vi "FGV_DOCK_REPORT_records_display.vi"(7 "options":T1, 8 "error_in":errorcluster, 11 "input":variant) -> (0 "error_out":errorcluster, 3 "output":variant)   [LabVIEW 2019]
uses:
  FGV_DOCK_REPORT_records_display.ctl
  DOCK_REPORT_references.ctl
  DOCK_REPORT_all_info.ctl
  SQL_CLIENT/MAIN/REPORTS/DATES/typedef/REPORT_DATES_statuses.ctl
  _misc/AULocalize/SubVIs/Get Localized Phrase Compact Interface 1D.vi
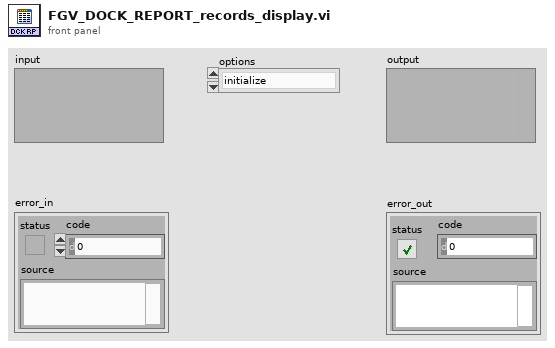
[diagram p1: front panel]
types:
  T1 = typedef "FGV_DOCK_REPORT_records_display.ctl" = enum16{"initialize", "set_cbatch_code", "set_records", "display", "clear", "get_all_info"}
  T2 = typedef "DOCK_REPORT_all_info.ctl" = cluster{"batch_code":string, "records":string[][], "record_statuses":T3[], "column_headers":string[], "column_widths":i16[], "DOCK_REPORT_references":T4}
  T3 = typedef "REPORT_DATES_statuses.ctl" = enum16{"GEAR_OK", "GEAR_NOK", "GEAR_interrupted", "GEAR_in_operation", "GEAR_unexpected"}
  T4 = typedef "DOCK_REPORT_references.ctl" = cluster{"front_panel_reference":refnum<vi>, "SQL_listbox_reference":refnum<vi>}
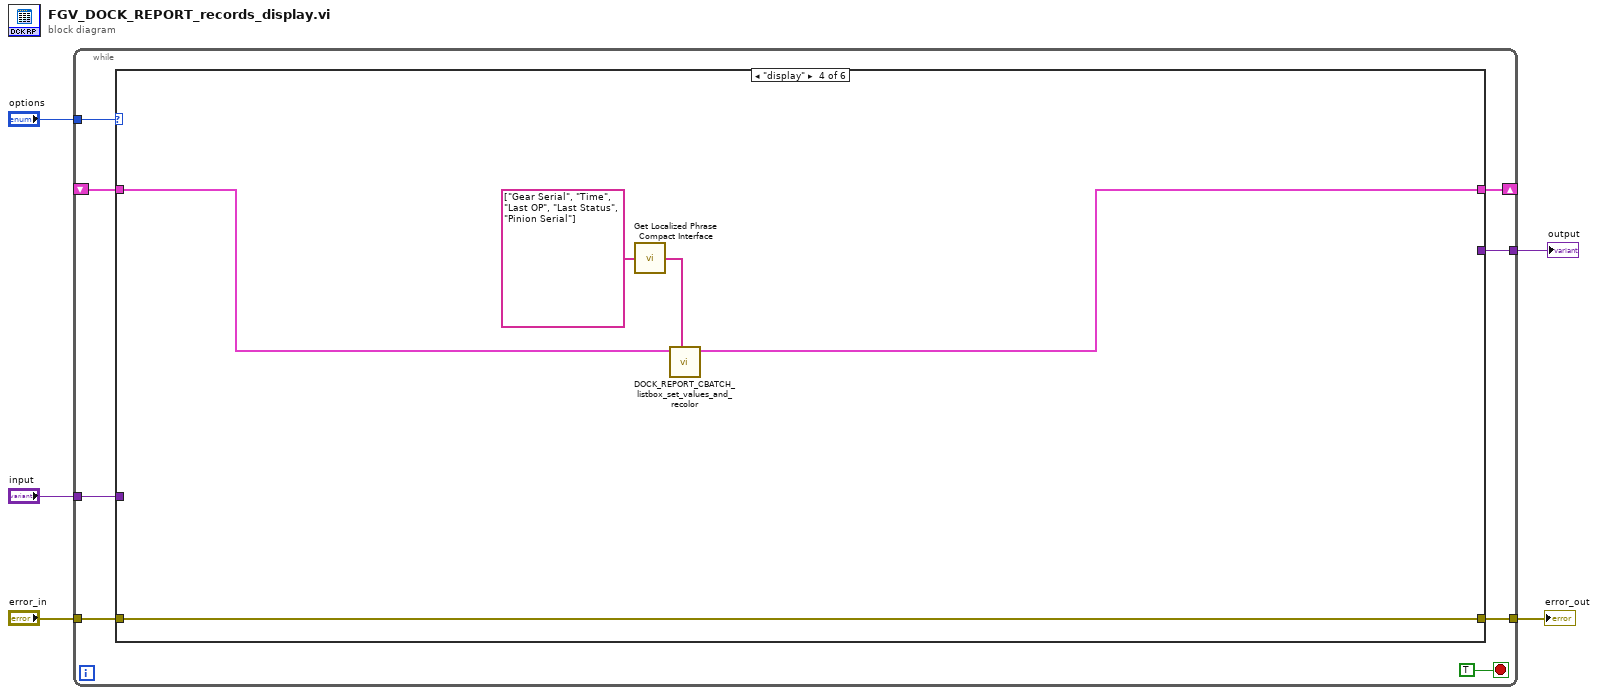
[diagram p0: block diagram]
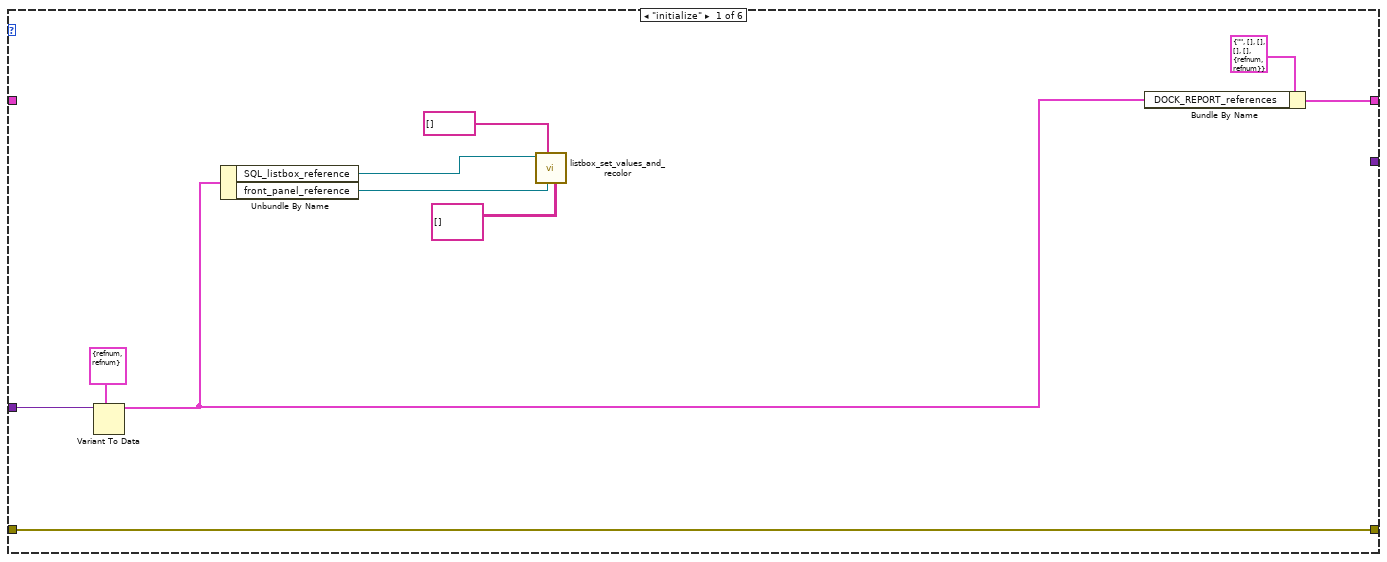
[diagram p2: hidden frame]
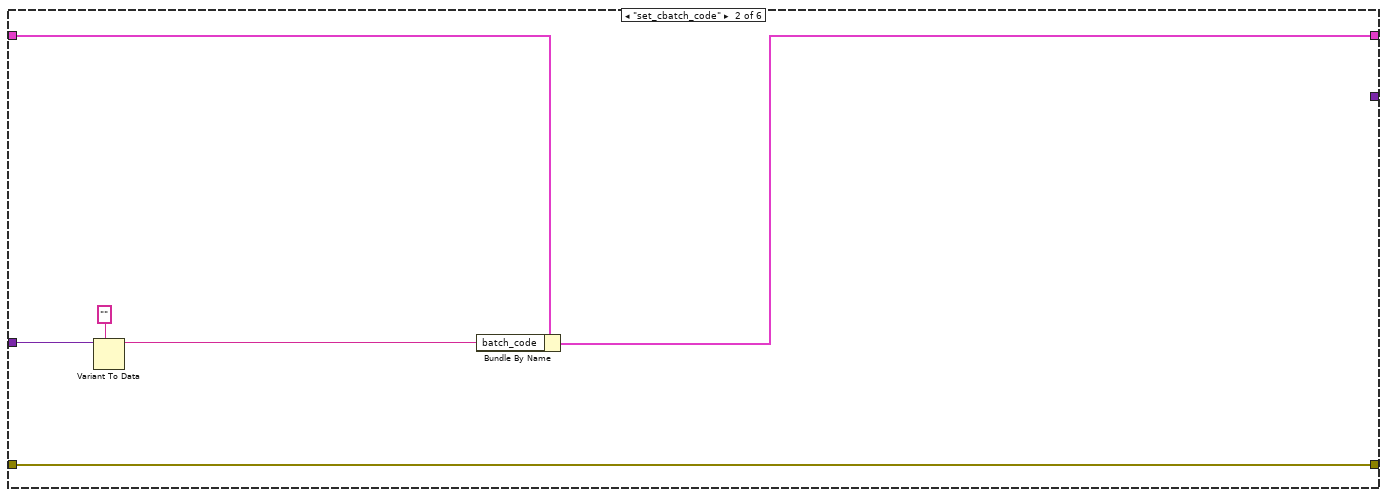
[diagram p3: hidden frame]
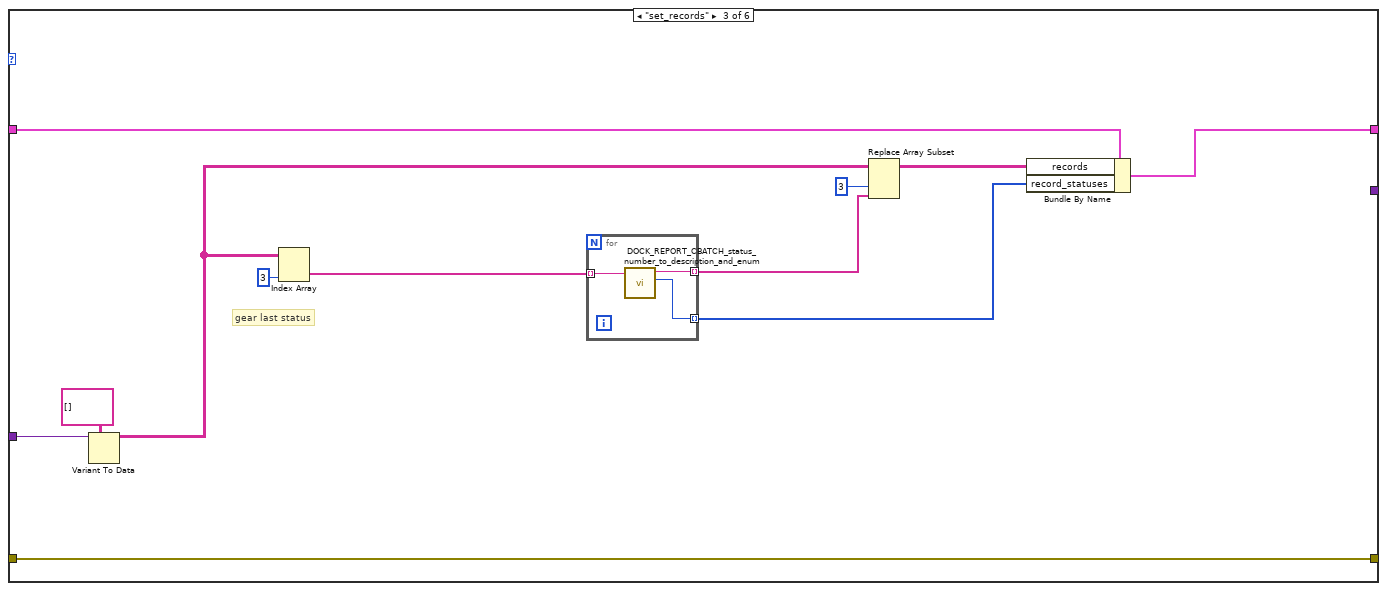
[diagram p4: hidden frame]
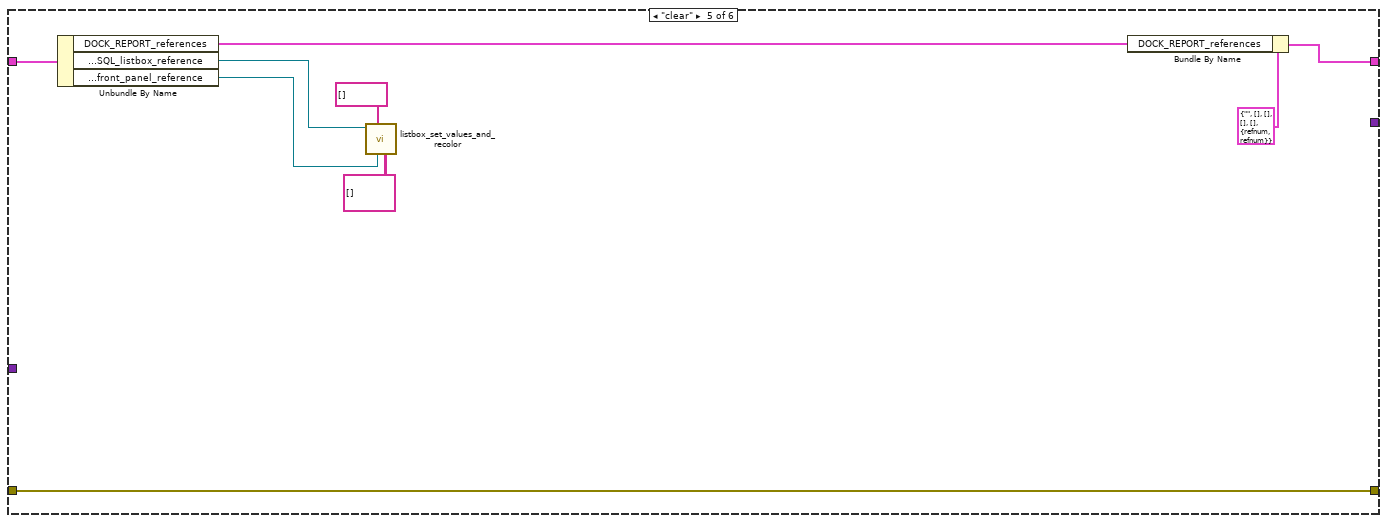
[diagram p5: hidden frame]
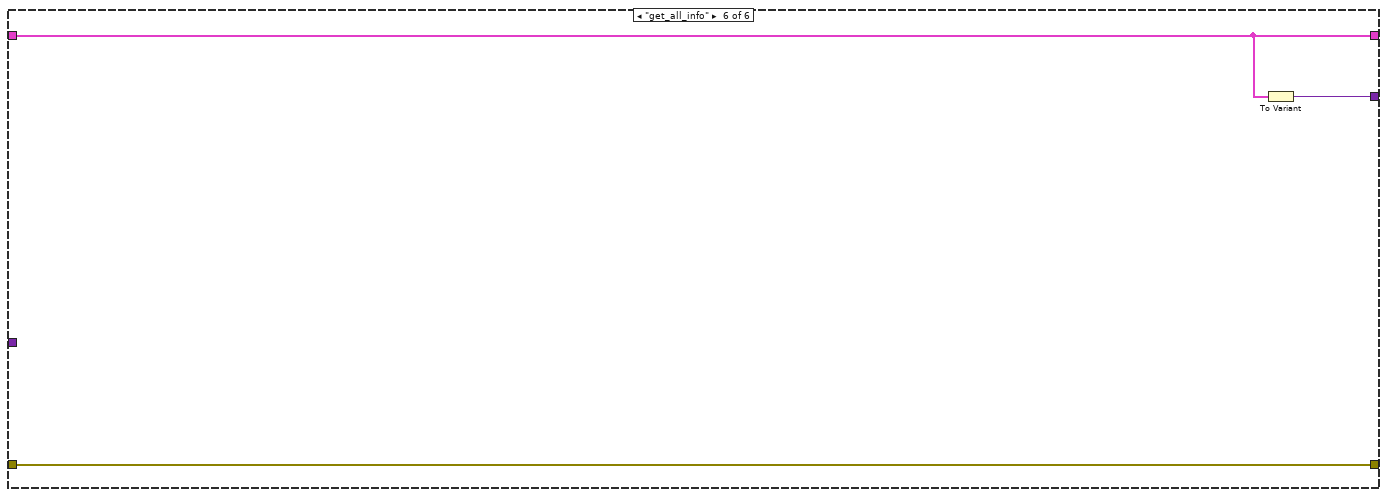
[diagram p6: hidden frame]
diagram:
  n1 = while {
    tunnel: "options" -> [w12]
    tunnel: [w11] -> w5
    tunnel: "error_in" -> [w10]
    shift-right: [w9] -> _
    shift-left: _ -> [w8]
    tunnel: "input" -> [w7]
    tunnel: [w6] -> w1
    stop <- TRUE stop-if-true
    n2 = case shown="\"display\"" w12 {
      tunnel: [w23 w24 w30 w49 w58 w61] -> w11
      tunnel: w10 -> [w23 w24 w30 w49 w58 w61]
      tunnel: [w15 w25 w31 w46 w52 w59] -> w9
      tunnel: w8 -> [_ w26 w32 w47 w55 w59]
      tunnel: w7 -> [w19 w27 w33 _ _ _]
      tunnel: [_ _ _ _ _ w60] -> w6
      frame "initialize" {
        n3 = Variant To Data(type=T4 {"front_panel_reference"=refnum, "SQL_listbox_reference"=refnum} ("REWORK_references"), Variant=w19) -> (data=w16:T4)  [unwired: 1 in, 1 out]
        n4 = Unbundle By Name(w16) -> ("SQL_listbox_reference"=w17:refnum<vi>, "front_panel_reference"=w18:refnum<vi>)
        n5 = call "listbox_set_values_and_recolor.vi"("item_names"=string[][] [], "front_panel_reference"=w18, "column_names"=string[] [], "multicolumn_listbox_reference_in"=w17) -> ()  [unwired: 6 in, 2 out]
        n6 = Bundle By Name(cluster=T2 {"batch_code"="", "records"=[], "record_statuses"=[], "column_headers"=[], "column_widths"=[], "DOCK_REPORT_references"={"front_panel_reference"=refnum, "SQL_listbox_reference"=refnum}} ("REPORT_all_info"), "DOCK_REPORT_references"=w16) -> (w15:T2)
      }
      frame "set_cbatch_code" {
        n7 = Variant To Data(type="", Variant=w27) -> (data=w28:string)  [unwired: 1 in, 1 out]
        n8 = Bundle By Name(cluster=w26, "batch_code"=w28) -> (w25:T2)
      }
      frame "set_records" {
        # "gear last status"
        n9 = Variant To Data(type=string[][] [], Variant=w33) -> (data=w37:string[][])  [unwired: 1 in, 1 out]
        n10 = Index Array(array=w37, index (col)=3 ("disabled index (col)")) -> (element=w39:string[])  [unwired: 1 in]
        n11 = for {
          tunnel: w39 -> [w44] mode=indexing
          tunnel: [w43] -> w38 mode=indexing
          tunnel: [w42] -> w34 mode=indexing
          n12 = call "DOCK_REPORT_CBATCH_status_number_to_description_and_enum.vi"("status_nmb"=w44) -> ("status_enum"=w43:T3, "status_description"=w42:string)  [unwired: 9 in]
        }
        n13 = Replace Array Subset(array=w37, new element=w34, index (col)=3 ("disabled index (col)")) -> (w35:string[][])  [unwired: 1 in]
        n14 = Bundle By Name(cluster=w32, "records"=w35, "record_statuses"=w38) -> (w31:T2)
      }
      frame "display" {
        n15 = call-poly "Get Localized Phrase Compact Interface.vi"("Key"=string[] ["Gear Serial", "Time", "Last OP", "Last Status", "Pinion Serial"] ("column_names")) -> ("Translated Phrase"=w45:string[])
        n16 = call "DOCK_REPORT_CBATCH_listbox_set_values_and_recolor.vi"("column_names"=w45, "REPORT_all_info_in"=w47) -> ("REPORT_all_info_out"=w46:T2)  [unwired: 8 in, 1 out]
      }
      frame "clear" {
        n17 = Unbundle By Name(w55) -> ("DOCK_REPORT_references"=w50:T4, "DOCK_REPORT_references.SQL_listbox_reference"=w54:refnum<vi>, "DOCK_REPORT_references.front_panel_reference"=w53:refnum<vi>)
        n18 = call "listbox_set_values_and_recolor.vi"("item_names"=string[][] [], "front_panel_reference"=w53, "column_names"=string[] [], "multicolumn_listbox_reference_in"=w54) -> ()  [unwired: 6 in, 2 out]
        n19 = Bundle By Name(cluster=T2 {"batch_code"="", "records"=[], "record_statuses"=[], "column_headers"=[], "column_widths"=[], "DOCK_REPORT_references"={"front_panel_reference"=refnum, "SQL_listbox_reference"=refnum}} ("REPORT_all_info"), "DOCK_REPORT_references"=w50) -> (w52:T2)
      }
      frame "get_all_info" {
        n20 = To Variant(anything=w59) -> (Variant=w60:variant)
      }
    }
  }
  "error_out" <- w5
  "output" <- w1
